vi "sub vi - AI USB4704 (3) v4.vi"() -> (1 "Graph 1":dynamicdata(graph), 2 "Graph 2":dynamicdata(graph), 3 "Graph 3":dynamicdata(graph), 4 "RMS values 1":dbl[](array[numeric]), 6 "RMS values 2":dbl[](array[numeric]), 8 "RMS values 3":dbl[](array[numeric]), 10 "loop time":dbl format="%.6g", 15 "error out":errorcluster)   [LabVIEW 2013]
uses:
  <vilib>/addons/Electrical Power/Basic/Measurement/RMS (N Channels).vi
  <vilib>/addons/Electrical Power/Basic/NI_EP_Basic.lvlib
panel:
  in  "Tab Control":enum32{"Page 1", "Page 2", "Page 3"}(tab)
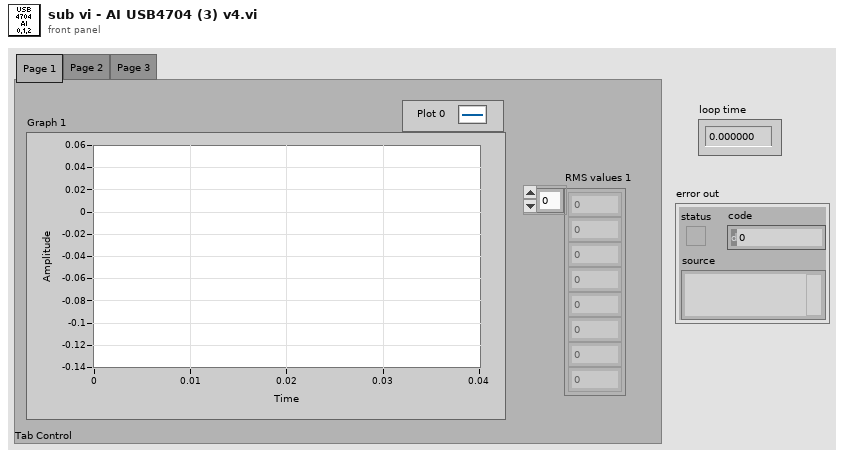
[diagram p1: front panel]
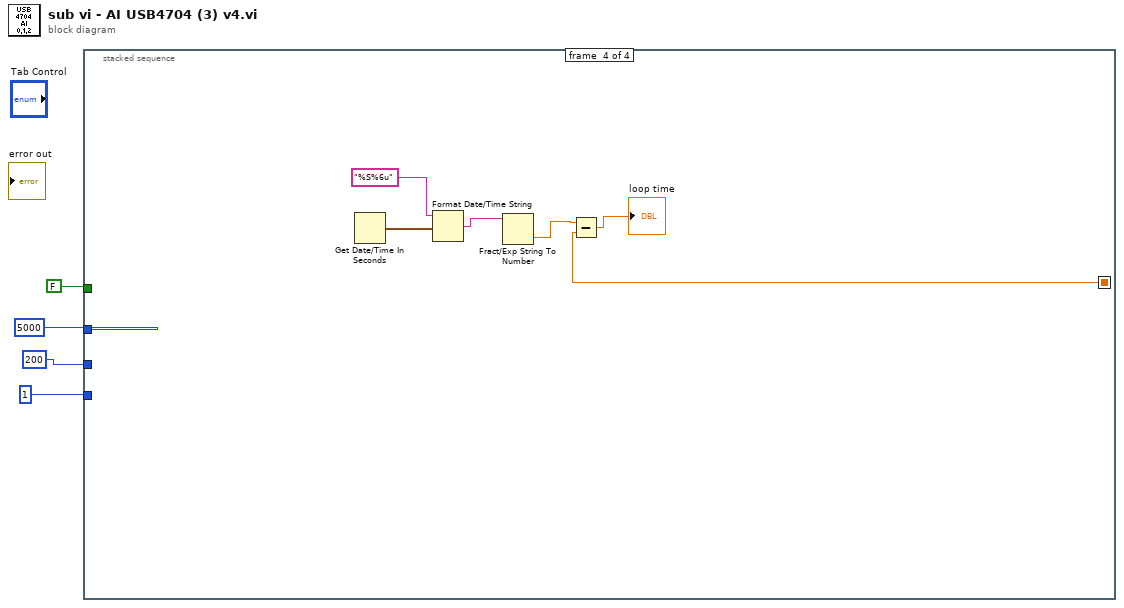
[diagram p0: block diagram]
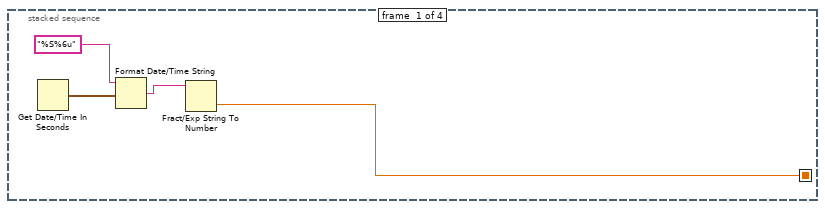
[diagram p2: hidden frame]
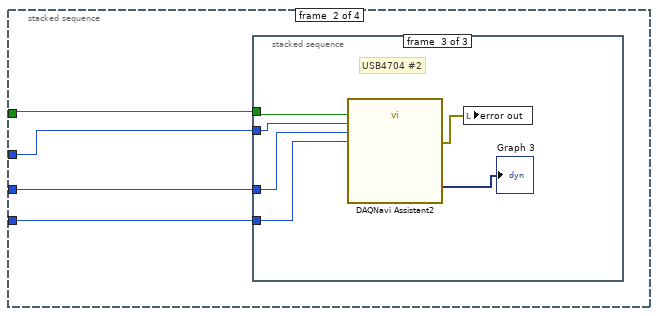
[diagram p3: hidden frame]
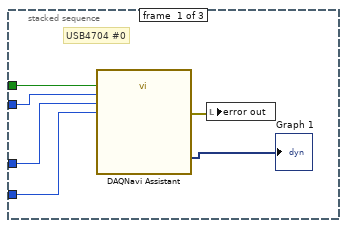
[diagram p4: hidden frame]
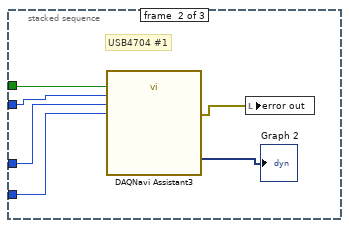
[diagram p5: hidden frame]
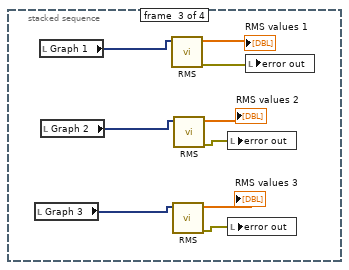
[diagram p6: hidden frame]
diagram:
  n1 = stacked-sequence {
    seq-local: [w5 _ _ _] -> [_ _ _ w41]
    tunnel: FALSE -> [_ w12 _ _]
    tunnel: 1 -> [_ w9 _ _]
    tunnel: 5000 -> [_ w11 _ _]
    tunnel: 200 -> [_ w10 _ _]
    frame #0 {
      n2 = Get Date/Time In Seconds() -> (seconds since 1Jan1904=w7:timestamp)
      n3 = Format Date/Time String(time format string (%c)="%S%6u", seconds (now)=w7) -> (date/time string=w6:string)  [unwired: 1 in]
      n4 = Fract/Exp String To Number(string=w6) -> (number=w5:dbl)  [unwired: 3 in, 1 out]
    }
    frame #1 {
      n5 = stacked-sequence {
        tunnel: w12 -> [w16 w23 w29]
        tunnel: w11 -> [w15 w22 w28]
        tunnel: w10 -> [w14 w21 w27]
        tunnel: w9 -> [w13 w20 w26]
        frame #0 {
          # "USB4704 #0"
          n6 = call "DAQNavi Assistant"("stop(true)"=w16, "conversion rate(Hz)"=w15, "samples"=w14, "time out(10s)"=w13) -> ("error out"=w17:errorcluster, "data out(DDT)"=→"Graph 1":dynamicdata)  [unwired: 22 in]
          n7 = local write "error out"(w17) -> ()
        }
        frame #1 {
          # "USB4704 #1"
          n8 = call "DAQNavi Assistant3"("stop(true)"=w23, "conversion rate(Hz)"=w22, "samples"=w21, "time out(10s)"=w20) -> ("error out"=w24:errorcluster, "data out(DDT)"=→"Graph 2":dynamicdata)  [unwired: 22 in]
          n9 = local write "error out"(w24) -> ()
        }
        frame #2 {
          # "USB4704 #2"
          n10 = call "DAQNavi Assistant2"("stop(true)"=w29, "conversion rate(Hz)"=w28, "samples"=w27, "time out(10s)"=w26) -> ("error out"=w30:errorcluster, "data out(DDT)"=→"Graph 3":dynamicdata)  [unwired: 22 in]
          n11 = local write "error out"(w30) -> ()
        }
      }
    }
    frame #2 {
      n12 = local read "Graph 3"() -> (w33:dynamicdata)
      n13 = local read "Graph 1"() -> (w39:dynamicdata)
      n14 = local read "Graph 2"() -> (w36:dynamicdata)
      n15 = call-poly <vilib>:"RMS.vi"("waveforms"=w39) -> ("error out"=w38:errorcluster, "RMS values"=→"RMS values 1":dbl[])  [unwired: 9 in]
      n16 = call-poly <vilib>:"RMS.vi"("waveforms"=w33) -> ("error out"=w32:errorcluster, "RMS values"=→"RMS values 3":dbl[])  [unwired: 9 in]
      n17 = call-poly <vilib>:"RMS.vi"("waveforms"=w36) -> ("error out"=w35:errorcluster, "RMS values"=→"RMS values 2":dbl[])  [unwired: 9 in]
      n18 = local write "error out"(w35) -> ()
      n19 = local write "error out"(w32) -> ()
      n20 = local write "error out"(w38) -> ()
    }
    frame #3 {
      n21 = Get Date/Time In Seconds() -> (seconds since 1Jan1904=w44:timestamp)
      n22 = Format Date/Time String(time format string (%c)="%S%6u", seconds (now)=w44) -> (date/time string=w43:string)  [unwired: 1 in]
      n23 = Fract/Exp String To Number(string=w43) -> (number=w42:dbl)  [unwired: 3 in, 1 out]
      n24 = Subtract(x=w42, y=w41) -> (x-y=→"loop time":dbl)
    }
  }
